vi "LinkBudget.vi"(0 "distance (km)":dbl format="%#_13g", 1 "Uplink frequency (GHz)":dbl format="%#_13g", 2 "Downlink frequency (GHz)":dbl format="%#_13g", 3 "Bandwith (MHz)":dbl, 4 "EIRPsat(dBW)":dbl format="%#_13g", 5 "EIRPground (dBW)":dbl format="%#_13g", 6 "G/Tsat (dB)":dbl format="%#_13g", 7 "G/T ground (dBK-1)":dbl format="%#_13g") -> (14 "C/N0 downlink (dBHz)":dbl format="%#_13g", 15 "C/N0 uplink (dBHz)":dbl format="%#_13g", 16 "C/N0 tot (dB)":dbl format="%#_13g", 17 "C/N (dB)":dbl)   [LabVIEW 2015]
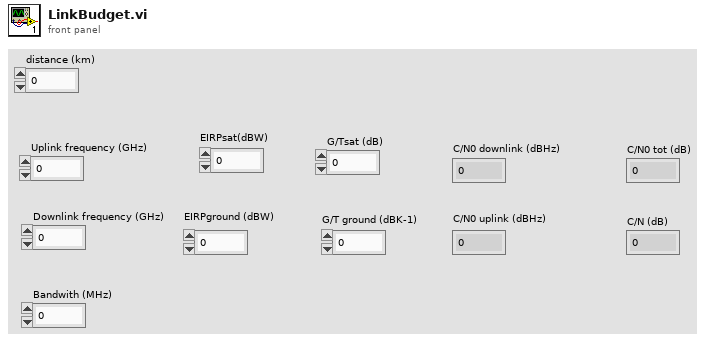
[diagram p1: front panel]
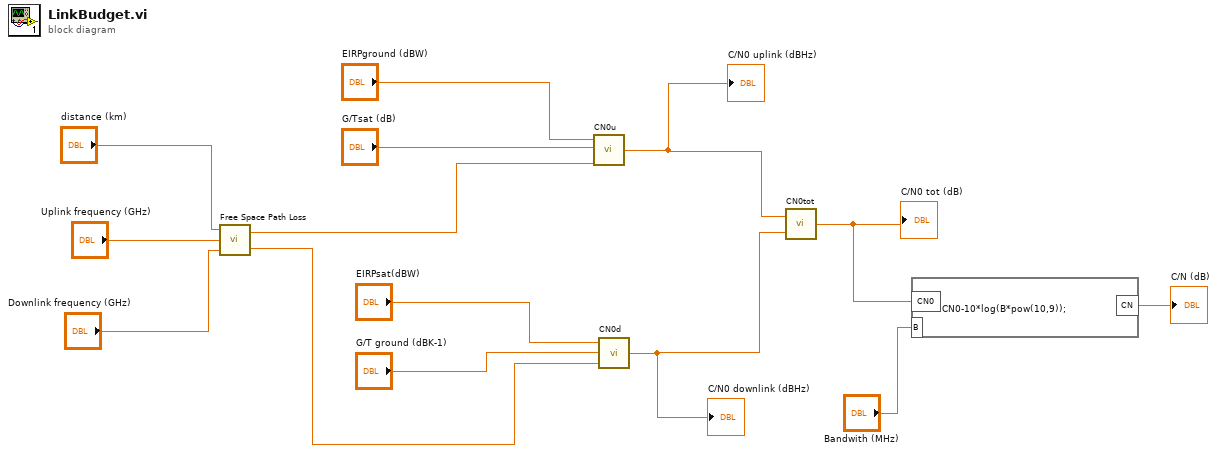
[diagram p0: block diagram]
diagram:
  n1 = call "Free Space Path Loss.vi"("Uplink Frequency (MHz)"="Downlink frequency (GHz)", "Downlink Frequency (MHz)"="Uplink frequency (GHz)", "distance (km)"="distance (km)") -> ("Downlink Free Space Path Loss (dB)"=w8:dbl, "Uplink Free Space Path Loss (dB)"=w11:dbl)
  n2 = call "CN0u.vi"("Uplink free space path loss (dB)"=w11, "G/Tsat (dBK-1)"="G/Tsat (dB)", "EIRP ground (dBW)"="EIRPground (dBW)") -> ("C/N0 uplink (dBHz)"=w4:dbl)
  "C/N0 uplink (dBHz)" <- w4
  n3 = call "CN0d.vi"("Downlink Free Space path Loss  (dB)"=w8, "G/T ground (dBK-1)"="G/T ground (dBK-1)", "EIRP sat (dBW)"="EIRPsat(dBW)") -> ("C/N0d (dBHz)"=w5:dbl)
  "C/N0 downlink (dBHz)" <- w5
  n4 = call "CN0tot.vi"("C/N0d (dBHz)"=w5, "C/N0u (dBHz)"=w4) -> ("C/N0tot (dBHz)"=w3:dbl)
  "C/N0 tot (dB)" <- w3
  n5 = formula code="CN=CN0-10*log(B*pow(10,9));"("CN0"=w3, "B"="Bandwith (MHz)") -> ("CN"=→"C/N (dB)":dbl)
